vi "FG Robot Status.vi"(2 "FG Action":T2, 3 "Status in":T1) -> (1 "Status out":T1)   [LabVIEW 2009]
uses:
  cRIO/Functional Global Variables/Actions for FG's.ctl
  Robot Status.ctl
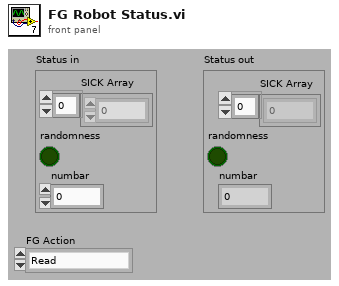
[diagram p1: front panel]
types:
  T1 = typedef "Robot Status.ctl" = cluster{"SICK Array":dbl[], "randomness":bool, "numbar":dbl}
  T2 = typedef "Actions for FG's.ctl" = enum16{"Read", "Write"}
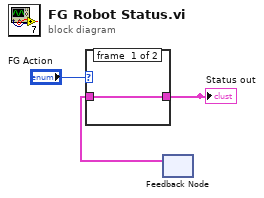
[diagram p0: block diagram]
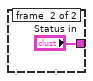
[diagram p2: hidden frame]
diagram:
  n1 = feedback #1() -> (w2:T1)  [unwired: 1 in]
  n2 = case shown="\"Read\", Default" "FG Action" {
    tunnel: [w4 "Status in"] -> w1
    tunnel: w2 -> [w4 _]
    frame #0 {
    }
    frame #1 {
    }
  }
  "Status out" <- w1
